vi "TraverseControl.vi"(0 "Mode":T1=enum."Read traverse position", 1 "Route Checking?":bool, 3 "Traverse Name":string, 7 "Model       Roll      Pitch       Yaw (deg)":dbl[](array[numeric]) format="%#.2f", 11 "Position input XYZ":dbl[](array[numeric])=[0.0, 0.0, 0.0] format="%.2f", 13 "Speed Factor":dbl=1.0 min=0.1 max=5.0 format="%.2f", 14 "Backlash Compensation?":bool=TRUE) -> (4 "Position Output XYZ":dbl[](array[numeric]) format="%.2f", 15 "Error String":string)   [LabVIEW 2011]
uses:
  Anemometry/Anemometry Sub Vis/Gen Trav/Trav_mode.ctl
  ~subVIs/GenericDriveCommand.ctl
  ADAM Client/Sub VIs/ADAM Controls/Update_scan_value.ctl
  Anemometry/Anemometry Sub Vis/Globals/Trav_pos_global.vi
  Anemometry/Anemometry Sub Vis/Globals/Preference_global.vi
  ~subVIs/DriveConfigGlobal.vi
  Anemometry/Anemometry Sub Vis/Gen Trav/Route mapping/Route_mapping_global.vi
panel:
  out "Server copy Location":path
  out "Position Steps":dbl[][](array[numeric]) format="%.2f"
  out "Log File":path
  out "Achieved Pos In Eng units of all channels":dbl[](array[numeric]) format="%.2f"
  out "Pulses Positon all channels":dbl[](array[numeric])
  out "Counters Reset?":bool
  # "X                Y                   Z"
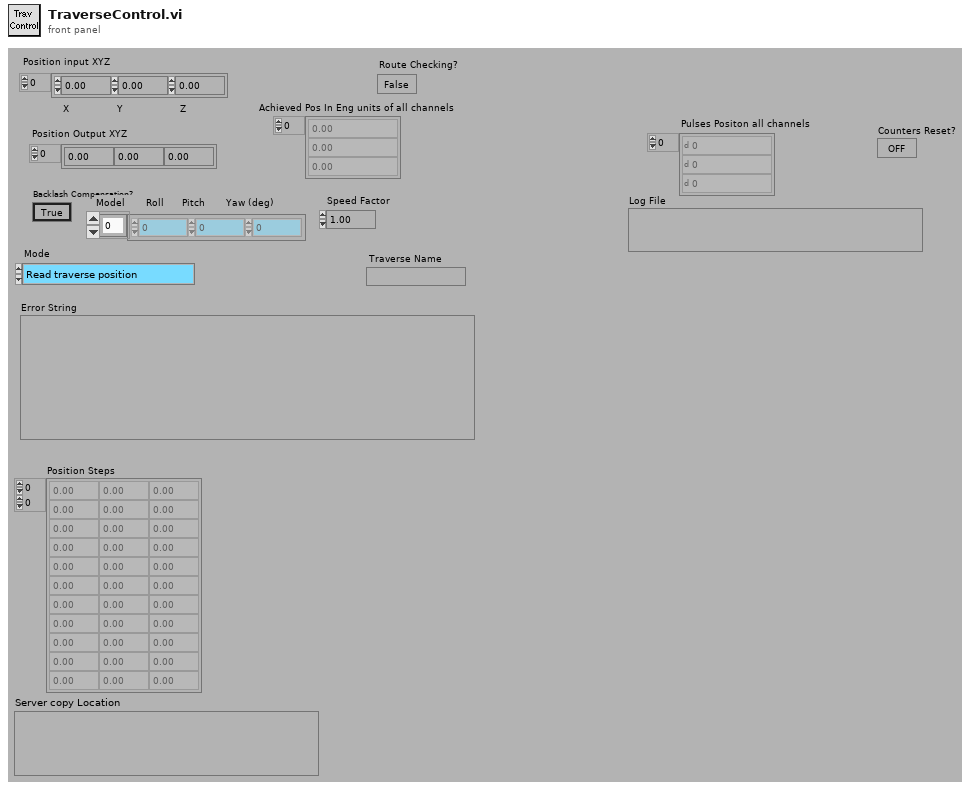
[diagram p1: front panel]
types:
  T1 = typedef "Trav_mode.ctl" = enum16{"Move traverse", "Read traverse position", "Teach Position"}
  T2 = typedef "Tunnel_Coordinates.ctl" = enum16{"Work in Tunnel Coordinates", "Work in Model Coordinates"}
  T3 = typedef "GenericDriveCommand.ctl" = string
  T4 = enum16{"To Traverse Coordinates", "To User Coordinates"}
  T5 = typedef "Update_scan_value.ctl" = cluster{"Channel Name":string, "New Value":dbl}
  T6 = typedef "AxisConfigCluster.ctl" = cluster{"Channel Properties":T7, "Static Drive Configuration":T8}
  T7 = typedef "DriveProperties.ctl" = cluster{"Channel Name":string, "Vel. Default":dbl, "Acc. Default":dbl, "Vel. Max":dbl, "Vel. Min":dbl, "Acc. Max":dbl, "Acc. Min":dbl, "Pulses/unit":dbl, "Address":u8, "Pulse Offset":i32, "Pos Tolerance":dbl, "Pulses/rev":dbl, "Backlash/Eng units":dbl, "Current Pos":dbl, "Ch Status":enum16{"Active", "Offline", "Simulate"}, "Port Name":string, "Axis Transform mode":string, "Metadata Ch Name":string, "Type":string}
  T8 = typedef "DriveStaticConfig.ctl" = cluster{"Correction Gain % (CG)":u16, "Dead Band (DB)":i32, "Dead Band Window (DW)":i32, "Encoder Resolution (ER)":i32, "Step Mode  (FSB)":u16, "Position Maintenance (FSC)":u16, "Stop on Stall (FSD)":u16, "Activate OP1 on stall (FSE)":u16, "Stop on Trigger 3 (FSF)":u16, "OP2 in Deadband (FSG)":u16, "Stall Detect (FSH)":u16, "Limit Disable (LD)":u16, "Motor Resolution (MR)":enum16{"200", "400", "1000", "2000", "4000", "5000", "10000", "12800", "18000", "20000", "21600", "25000", "25400", "25600", "36000", "50000", "278528", "425984", "507904", "614400", "655360", "819200", "1024000"}, "Limit Switch Sense (OSA)":u16, "Home Position (OSB)":u16, "Home Switch Sense (OSC)":u16, "Encoder Z for Home (OSD)":u16, "Reference edge of Home (OSH)":u16, "RS232 Echo Control (SSA)":u16, "Buffer at Limit (SSG)":u16, "Buffer at Stop (SSH)":u16, "Indexer Mode  (FSA)":u16, "Type":string, "ConfigString":string, "De Power Motor":enum16{"TRUE", "FALSE"}}
  T9 = typedef "Box_size.ctl" = cluster{"Max":dbl, "Min":dbl}[]
  T10 = typedef "Exclude_cluster.ctl" = cluster{"Sizes":T9, "Name":string, "Exclude Type":T11}
  T11 = typedef "Exclusion_type.ctl" = enum16{"Exclude completely", "Allow only vertical moves"}
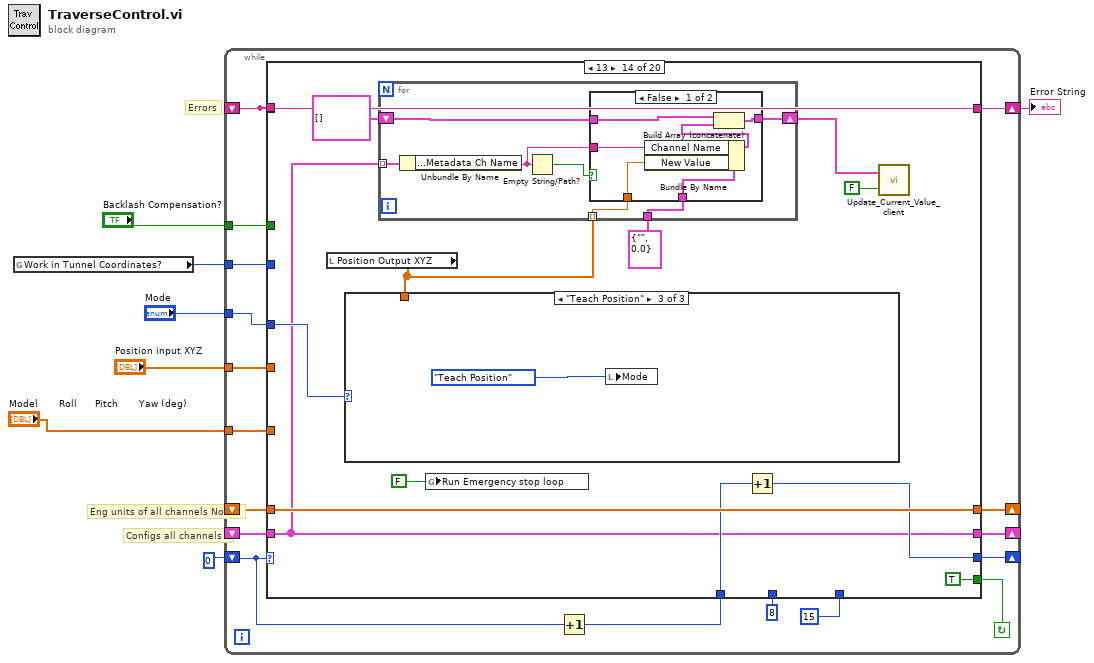
[diagram p0: block diagram]
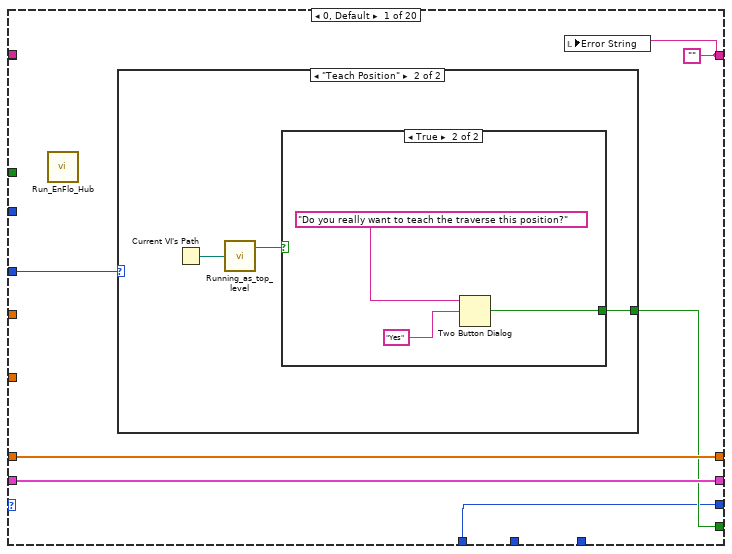
[diagram p2: hidden frame]
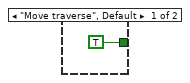
[diagram p3: hidden frame]
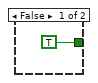
[diagram p4: hidden frame]
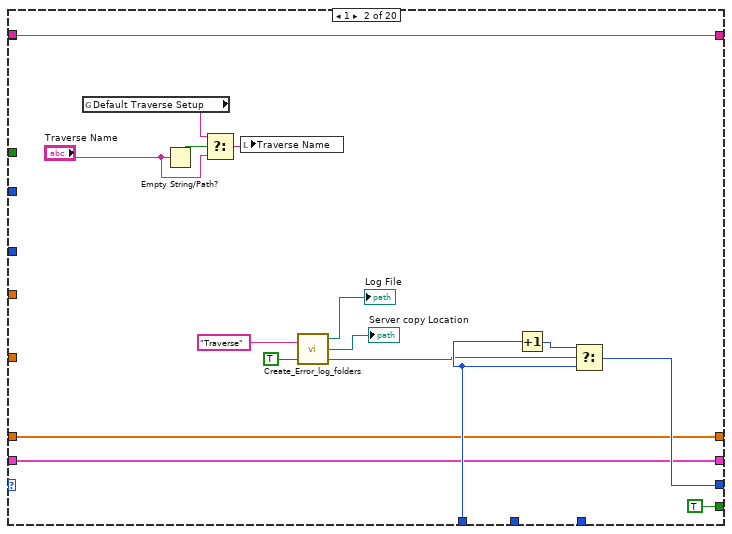
[diagram p5: hidden frame]
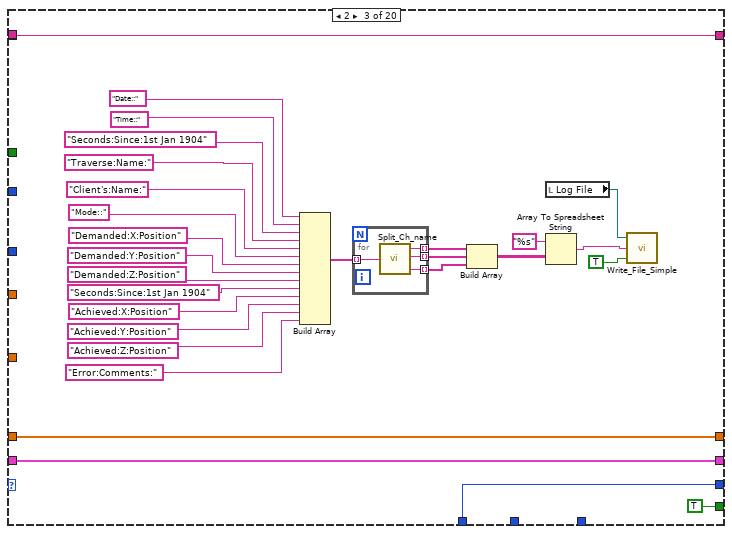
[diagram p6: hidden frame]
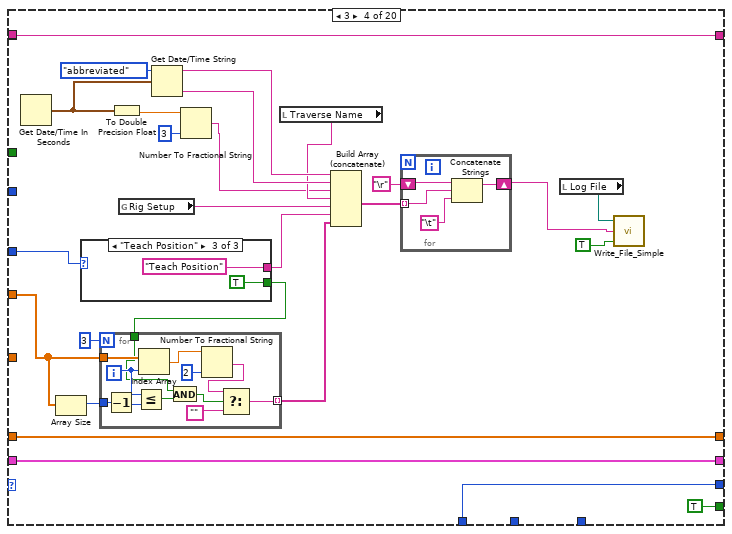
[diagram p7: hidden frame]
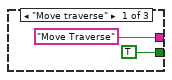
[diagram p8: hidden frame]
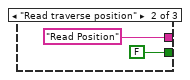
[diagram p9: hidden frame]
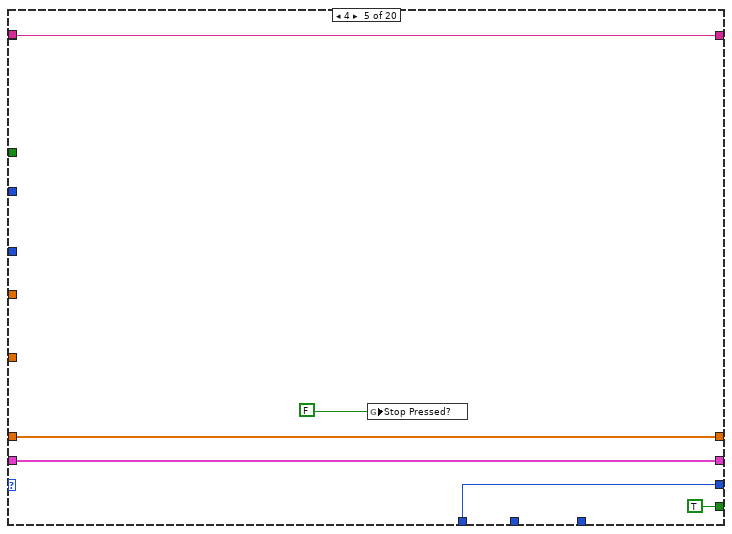
[diagram p10: hidden frame]
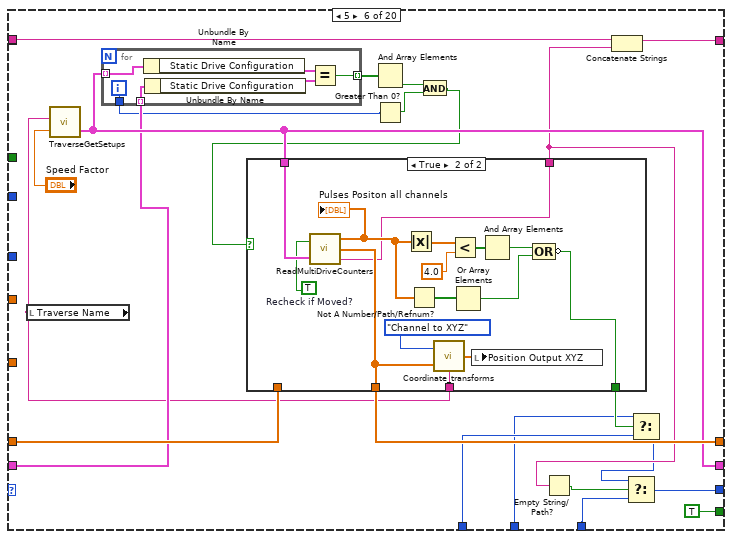
[diagram p11: hidden frame]
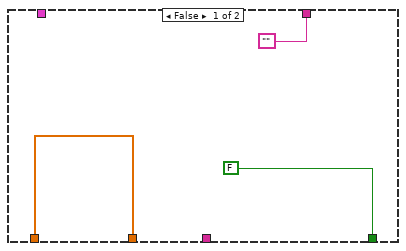
[diagram p12: hidden frame]
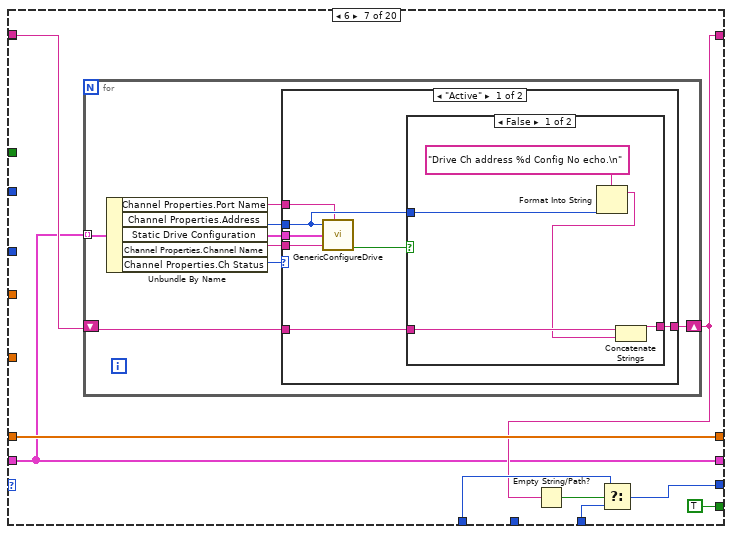
[diagram p13: hidden frame]
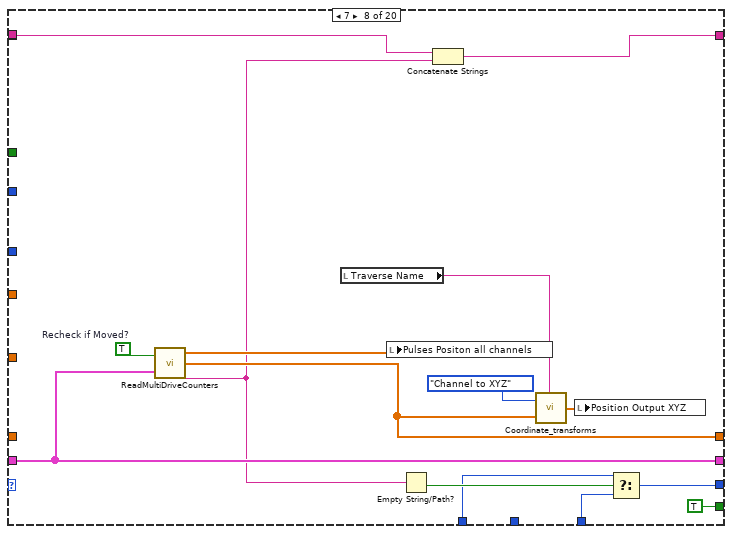
[diagram p16: hidden frame]
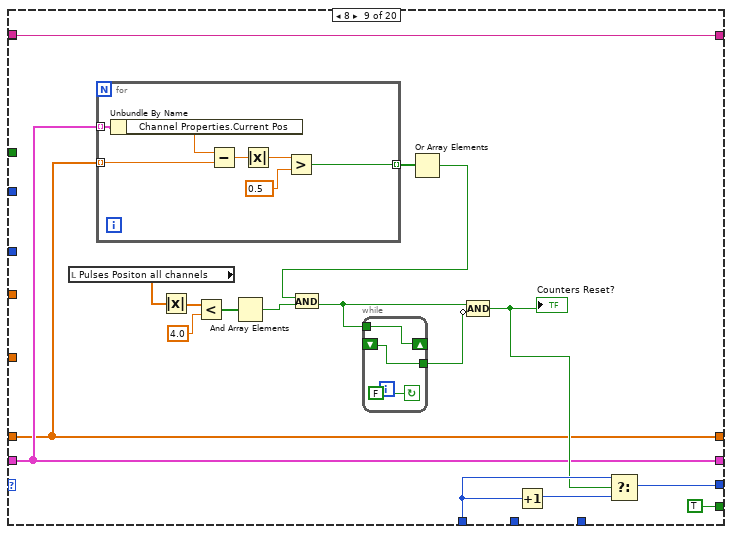
[diagram p17: hidden frame]
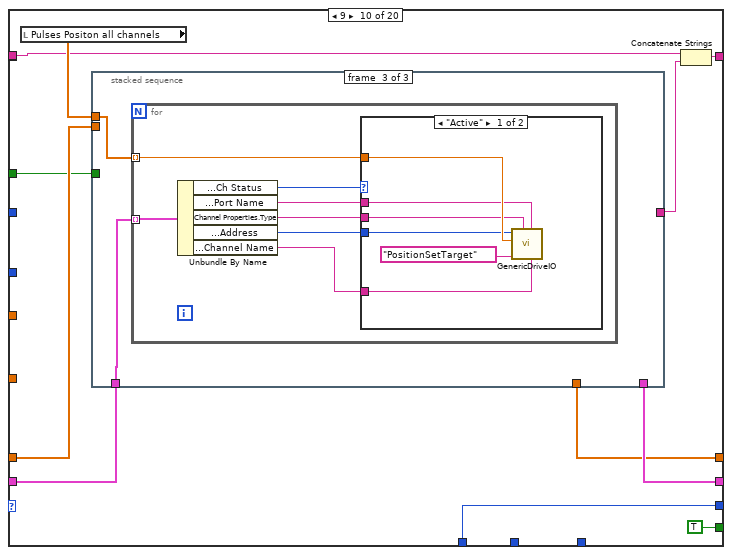
[diagram p18: hidden frame]
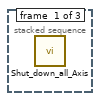
[diagram p19: hidden frame]
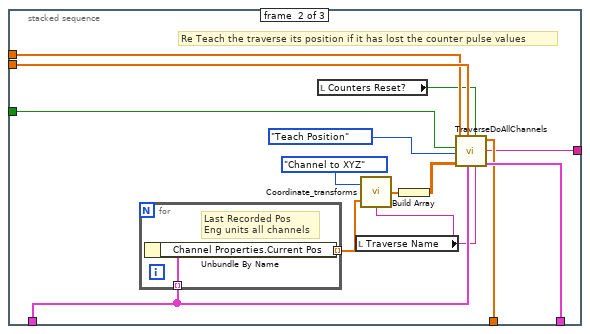
[diagram p20: hidden frame]
diagram:
  # "Errors"
  # "Eng units of all channels Now"
  # "Configs all channels"
  n1 = global read "Trav_pos_global.vi" "Work in Tunnel Coordinates?"() -> (w2:T2)
  n2 = while {
    tunnel: "Backlash Compensation?" -> [w10]
    tunnel: "Position input XYZ" -> [w14]
    shift-left: _ -> [w11]
    shift-right: [w15] -> w5
    shift-left: _ -> [w16]
    shift-right: [w17] -> _
    shift-left: _ -> [w18]
    shift-right: [w19] -> _
    shift-left: 0 -> [w22]
    shift-right: [w20] -> _
    tunnel: "Mode" -> [w24]
    tunnel: "Model       Roll      Pitch       Yaw (deg)" -> [w9]
    tunnel: w2 -> [w8]
    stop <- w23 continue-if-true
    n3 = Increment(x=w22) -> (x+1=w21:i32)
    n4 = case shown="13" w22 {
      tunnel: w24 -> [w30 _ _ w105 _ _ _ _ _ _ w309 _ w373 w380 _ _ _ w453 _ w509]
      tunnel: [w27 TRUE ("T button?") TRUE ("T button?") TRUE ("T button?") TRUE TRUE ("T button?") TRUE ("T button?") TRUE ("T button?") TRUE TRUE TRUE ("T button?") TRUE ("T button?") TRUE TRUE TRUE ("T button?") TRUE ("T button?") TRUE ("T button?") w455 TRUE FALSE] -> w23
      tunnel: w21 -> [w26 w53 w62 w110 w135 w159 w192 w220 w245 w261 w308 w342 w364 w382 w405 w419 w448 w452 w487 w516]
      tunnel: [w26 w51 w62 w110 w135 w142 w191 w218 w243 w261 w307 w343 w364 w381 w405 w417 w448 w451 w487 w516] -> w20
      tunnel: [w28 w48 w64 w112 w137 w157 w187 w232 w239 w270 w305 w345 w357 w379 w407 w431 w450 w458 w485 w514] -> w19
      tunnel: w18 -> [w28 w48 w64 w112 w137 w156 w187 w232 w239 w269 w305 w345 w371 w379 w407 w431 w450 w458 w485 w514]
      tunnel: [w29 w49 w63 w111 w138 w162 w195 w227 w238 w266 w304 w332 w365 w385 w406 w430 w449 w459 w488 w517] -> w17
      tunnel: w16 -> [w29 w49 w63 w111 w138 w161 w195 _ w238 w267 w304 w332 w360 w385 w406 w430 w449 w459 w488 w517]
      tunnel: [w25 w47 w60 w102 w139 w147 w188 w223 w242 w263 w310 w336 w367 w383 w403 w421 w446 w454 w481 w510] -> w15
      tunnel: w11 -> [_ w47 w60 w102 w139 w148 w189 w224 w242 w265 w310 _ w368 w383 w403 w421 w446 w457 w483 w512]
      tunnel: w14 -> [_ _ _ w99 _ _ _ _ _ _ w303 w334 _ _ _ _ _ _ w479 _]
      tunnel: 15 ("f") -> [_ _ _ _ _ w143 w190 w219 _ _ _ w338 _ _ _ _ _ _ _ _]
      tunnel: 8 ("t") -> [_ _ _ _ _ w158 _ _ _ _ _ _ _ _ _ _ _ _ _ _]
      tunnel: w11 -> [_ _ _ _ _ _ _ _ _ _ _ w339 _ _ _ _ _ _ _ _]
      tunnel: w10 -> [_ _ _ _ _ _ _ _ _ w260 _ _ w359 _ _ _ _ _ _ _]
      tunnel: w9 -> [_ _ _ _ _ _ _ _ _ _ _ w319 _ _ _ _ _ _ w480 w507]
      tunnel: w8 -> [_ _ _ _ _ _ _ _ _ _ _ _ _ _ _ _ _ _ w477 w505]
      frame 0, Default {
        w25 = ""
        n5 = call "Run_EnFlo_Hub.vi"() -> ()  [unwired: 8 out]
        n6 = case shown="\"Teach Position\"" w30 {
          tunnel: [TRUE ("T button?") w32] -> w27
          frame "Move traverse", Default {
          }
          frame "Teach Position" {
            n7 = Current VI's Path() -> (path=w34:path)
            n8 = call "Running_as_top_level.vi"("Vi path name"=w34) -> ("Top Level"=w33:bool)  [unwired: 1 out]
            n9 = case shown="True" w33 {
              tunnel: [TRUE ("T button?") w36] -> w32
              frame False {
              }
              frame True {
                n10 = Two Button Dialog(message="Do you really want to teach the traverse this position?", 2:"Yes" ("T button name (\"OK\")")) -> (T button?=w36:bool)  [unwired: 1 out]
              }
            }
          }
        }
        n11 = local write "Error String"(w25) -> ()
      }
      frame 1 {
        n12 = global read "Trav_pos_global.vi" "Default Traverse Setup"() -> (w44:string)
        n13 = Empty String/Path?(string/path="Traverse Name") -> (empty?=w42:bool)
        n14 = Select(t=w44, s=w42, f="Traverse Name") -> (s? t:f=w41:string)
        n15 = local write "Traverse Name"(w41) -> ()
        n16 = call "Create_Error_log_folders.vi"("Per Day Log File?"=TRUE, "Log Filename"="Traverse" ("Input Element")) -> ("exists?"=w45:bool, "Server copy Location"=→"Server copy Location":path, "Local Log File"=→"Log File":path)  [unwired: 1 in]
        n17 = Increment(x=w53) -> (x+1=w52:i32)
        n18 = Select(t=w52, s=w45, f=w53) -> (s? t:f=w51:i32)
      }
      frame 2 {
        n19 = Build Array("Date::", "Time::", "Seconds:Since:1st Jan 1904", "Traverse:Name:", "Client's:Name:", "Mode::", "Demanded:X:Position", "Demanded:Y:Position", "Demanded:Z:Position", "Seconds:Since:1st Jan 1904", "Achieved:X:Position", "Achieved:Y:Position", "Achieved:Z:Position", "Error:Comments:") -> (w67:string[])
        n20 = for {
          tunnel: w67 -> [w86] mode=indexing
          tunnel: [w85] -> w68 mode=indexing
          tunnel: [w84] -> w69 mode=indexing
          tunnel: [w83] -> w70 mode=indexing
          n21 = call "Split_Ch_name.vi"("Ch name"=w86) -> ("Top level"=w85:string, "Middle"=w84:string, "Low level"=w83:string)
        }
        n22 = Build Array(w68, w69, w70) -> (w65:string[][])
        n23 = local read "Log File"() -> (w56:path)
        n24 = Array To Spreadsheet String(array=w65, 3:"%s" ("format string")) -> (spreadsheet string=w57:string)  [unwired: 1 out]
        n25 = call "Write_File_Simple.vi"("append to file? (new file:F)"=TRUE, "character string"=w57, "file path"=w56) -> ()  [unwired: 2 out]
      }
      frame 3 {
        n26 = Get Date/Time In Seconds() -> (seconds since 1Jan1904=w91:timestamp)
        n27 = Array Size(array=w99) -> (size(s)=w100:i32)
        n28 = case shown="\"Teach Position\"" w105 {
          tunnel: ["Move Traverse" "Read Position" "Teach Position"] -> w106
          tunnel: [TRUE FALSE TRUE] -> w96
          frame "Move traverse" {
          }
          frame "Read traverse position" {
          }
          frame "Teach Position" {
          }
        }
        n29 = for {
          N: 3 -> [_]
          tunnel: w99 -> [w124]
          tunnel: w100 -> [w121]
          tunnel: [w117] -> w97 mode=indexing
          tunnel: w96 -> [w113]
          i -> [w119]
          n30 = Decrement(x=w121) -> (x-1=w120:i32)
          n31 = Less Or Equal?(x=w119, y=w120) -> (x <= y?=w115:bool)
          n32 = Index Array(array=w124, index=w119) -> (element=w123:dbl)
          n33 = And(x=w113, y=w115) -> (x .and. y?=w114:bool)
          n34 = Number To Fractional String(number=w123, precision (6)=i16 2) -> (F-format string=w118:string)  [unwired: 2 out]
          n35 = Select(t=w118, s=w114, f="") -> (s? t:f=w117:string)
        }
        n36 = To Double Precision Float(number=w91) -> (double precision float=w90:dbl)
        n37 = global read "Preference_global.vi" "Rig Setup"() -> (w87:string)
        n38 = Get Date/Time String(date format (0)=enum16{"short", "long", "abbreviated"}."abbreviated", seconds (now)=w91) -> (date string=w108:string, time string=w107:string)  [unwired: 1 out]
        n39 = Number To Fractional String(number=w90, precision (6)=i16 3) -> (F-format string=w88:string)  [unwired: 2 out]
        n40 = local read "Traverse Name"() -> (w92:string)
        n41 = Build Array (concatenate)(w108, w107, w88, w92, w87, w106, w97) -> (w103:string[])
        n42 = for {
          shift-right: [w127] -> w93
          shift-left: "\r" -> [w128]
          tunnel: w103 -> [w126] mode=indexing
          n43 = Concatenate Strings(w128, w126, "\t") -> (w127:string)
        }
        n44 = local read "Log File"() -> (w94:path)
        n45 = call "Write_File_Simple.vi"("append to file? (new file:F)"=TRUE, "character string"=w93, "file path"=w94) -> ()  [unwired: 2 out]
      }
      frame 4 {
        n46 = global write "DriveConfigGlobal.vi" "Stop Pressed?"(FALSE) -> ()
      }
      frame 5 {
        n47 = local read "Traverse Name"() -> (w150:string)
        n48 = call "TraverseGetSetups.vi"("Speed Factor"="Speed Factor", "Traverse Name"=w150) -> ("Matched Configurations"=w157:T6[])  [unwired: 1 out]
        n49 = for {
          tunnel: w157 -> [w168] mode=indexing
          tunnel: w156 -> [w167] mode=indexing
          tunnel: [w164] -> w155 mode=indexing
          tunnel: [w163] -> w154
          i -> [w163]
          n50 = Unbundle By Name(w168) -> ("Static Drive Configuration"=w166:T8)
          n51 = Unbundle By Name(w167) -> ("Static Drive Configuration"=w165:T8)
          n52 = Equal?(x=w166, y=w165) -> (x = y?=w164:bool)
        }
        n53 = And Array Elements(Boolean array=w155) -> (logical AND=w152:bool)
        n54 = Greater Than 0?(x=w154) -> (x > 0?=w153:bool)
        n55 = And(x=w152, y=w153) -> (x .and. y?=w151:bool)
        n56 = case shown="True" w151 {
          tunnel: w157 -> [_ w186]
          tunnel: [w171 w176] -> w162
          tunnel: w161 -> [w171 _]
          tunnel: [FALSE w178] -> w160
          tunnel: w150 -> [_ w174]
          tunnel: ["" w172] -> w146
          frame False {
          }
          frame True {
            w173 = TRUE  # Recheck if Moved?
            n57 = call "ReadMultiDriveCounters.vi"("Recheck if Moved?"=w173, "Matched Configurations"=w186) -> ("Pulses"=w181:dbl[], "Eng units"=w176:dbl[], "Error String"=w172:string)
            "Pulses Positon all channels" <- w181
            n58 = Absolute Value(x=w181) -> (abs(x)=w185:dbl[])
            n59 = Not A Number/Path/Refnum?(number/path/refnum=w181) -> (NaN/Path/Refnum?=w180:bool[])
            n60 = call "Coordinate_transforms.vi"("Traverse Name"=w174, "Input"=w176, "Mode"=enum16{"XYZ to Channel", "Channel to XYZ"}."Channel to XYZ") -> ("Output"=w175:dbl[])
            n61 = Less?(x=w185, y=4.0 ("Achieved Position")) -> (x < y?=w183:bool[])
            n62 = Or Array Elements(Boolean array=w180) -> (logical OR=w179:bool)
            n63 = local write "Position Output XYZ"(w175) -> ()
            n64 = And Array Elements(Boolean array=w183) -> (logical AND=w182:bool)
            n65 = Compound Arithmetic op=OR(w182, w179) -> (invert w178:bool)
          }
        }
        n66 = Empty String/Path?(string/path=w146) -> (empty?=w145:bool)
        n67 = Concatenate Strings(w148, w146) -> (w147:string)
        n68 = Select(t=w158, s=w160, f=w159) -> (s? t:f=w144:i32)
        n69 = Select(t=w144, s=w145, f=w143) -> (s? t:f=w142:i32)
      }
      frame 6 {
        n70 = for {
          tunnel: w187 -> [w203] mode=indexing
          shift-right: [w196] -> w188
          shift-left: w189 -> [w197]
          n71 = Unbundle By Name(w203) -> ("Channel Properties.Port Name"=w198:string, "Channel Properties.Address"=w202:u8, "Static Drive Configuration"=w201:T8, "Channel Properties.Channel Name"=w200:string, "Channel Properties.Ch Status"=w199:enum16{"Active", "Offline", "Simulate"})
          n72 = case shown="\"Active\"" w199 {
            tunnel: w202 -> [w208 _]
            tunnel: w201 -> [w210 _]
            tunnel: w200 -> [w209 _]
            tunnel: w198 -> [w207 _]
            tunnel: w197 -> [w205 w217]
            tunnel: [w204 w217] -> w196
            frame "Active" {
              n73 = call "GenericConfigureDrive.vi"("Address"=w208, "Port Name"=w207, "Static Drive Configuration"=w210, "Channel Name"=w209) -> ("Good Echo"=w206:bool)  [unwired: 4 out]
              n74 = case shown="False" w206 {
                tunnel: w208 -> [w215 _]
                tunnel: w205 -> [w213 w216]
                tunnel: [w212 w216] -> w204
                frame False {
                  n75 = Format Into String(format string="Drive Ch address %d Config No echo.\n" ("Format String"), w215) -> (resulting string=w211:string)  [unwired: 2 in, 1 out]
                  n76 = Concatenate Strings(w213, w211) -> (w212:string)
                }
                frame True {
                }
              }
            }
            frame "Offline", Default {
            }
          }
        }
        n77 = Empty String/Path?(string/path=w188) -> (empty?=w193:bool)
        n78 = Select(t=w192, s=w193, f=w190) -> (s? t:f=w191:i32)
      }
      frame 7 {
        w225 = TRUE  # Recheck if Moved?
        n79 = call "ReadMultiDriveCounters.vi"("Recheck if Moved?"=w225, "Matched Configurations"=w232) -> ("Pulses"=w230:dbl[], "Eng units"=w227:dbl[], "Error String"=w221:string)
        n80 = local read "Traverse Name"() -> (w226:string)
        n81 = local write "Pulses Positon all channels"(w230) -> ()
        n82 = Empty String/Path?(string/path=w221) -> (empty?=w222:bool)
        n83 = Concatenate Strings(w224, w221) -> (w223:string)
        n84 = call "Coordinate_transforms.vi"("Traverse Name"=w226, "Input"=w227, "Mode"=enum16{"XYZ to Channel", "Channel to XYZ"}."Channel to XYZ") -> ("Output"=w228:dbl[])
        n85 = local write "Position Output XYZ"(w228) -> ()
        n86 = Select(t=w220, s=w222, f=w219) -> (s? t:f=w218:i32)
      }
      frame 8 {
        n87 = local read "Pulses Positon all channels"() -> (w233:dbl[])
        n88 = for {
          tunnel: w239 -> [w259] mode=indexing
          tunnel: w238 -> [w257] mode=indexing
          tunnel: [w253] -> w236 mode=indexing
          n89 = Unbundle By Name(w259) -> ("Channel Properties.Current Pos"=w258:dbl)
          n90 = Subtract(x=w258, y=w257) -> (x-y=w256:dbl)
          n91 = Absolute Value(x=w256) -> (abs(x)=w255:dbl)
          n92 = Greater?(x=w255, y=0.5) -> (0:w253:bool)
        }
        n93 = Absolute Value(x=w233) -> (abs(x)=w249:dbl[])
        n94 = Less?(x=w249, y=4.0 ("Achieved Position")) -> (x < y?=w247:bool[])
        n95 = And Array Elements(Boolean array=w247) -> (logical AND=w237:bool)
        n96 = Or Array Elements(Boolean array=w236) -> (logical OR=w235:bool)
        n97 = And(x=w235, y=w237) -> (x .and. y?=w234:bool)
        n98 = while {
          tunnel: [w251] -> w241
          tunnel: w234 -> [w252]
          shift-left: _ -> [w251]
          shift-right: [w252] -> _
          stop <- FALSE continue-if-true
        }
        n99 = Compound Arithmetic op=AND(w234, invert w241) -> (w240:bool)
        "Counters Reset?" <- w240
        n100 = Increment(x=w245) -> (x+1=w244:i32)
        n101 = Select(t=w245, s=w240, f=w244) -> (s? t:f=w243:i32)
      }
      frame 9 {
        n102 = local read "Pulses Positon all channels"() -> (w268:dbl[])
        n103 = stacked-sequence {
          tunnel: w268 -> [_ w276 w287]
          tunnel: [_ w284 _] -> w270
          tunnel: w267 -> [_ w283 _]
          tunnel: [_ w282 _] -> w266
          tunnel: w269 -> [_ w278 w288]
          tunnel: [_ w281 _] -> w264
          tunnel: w260 -> [_ w272 _]
          frame #0 {
            n104 = call "Shut_down_all_Axis.vi"() -> ()  [unwired: 1 out]
          }
          frame #1 {
            # "Re Teach the traverse its position if it has lost the counter pulse values"
            n105 = for {
              tunnel: [w286] -> w277 mode=indexing
              tunnel: w278 -> [w285] mode=indexing
              # "Last Recorded Pos\nEng units all channels"
              n106 = Unbundle By Name(w285) -> ("Channel Properties.Current Pos"=w286:dbl)
            }
            n107 = local read "Counters Reset?"() -> (w274:bool)
            n108 = local read "Traverse Name"() -> (w273:string)
            n109 = call "Coordinate_transforms.vi"("Traverse Name"=w273, "Input"=w277, "Mode"=enum16{"XYZ to Channel", "Channel to XYZ"}."Channel to XYZ") -> ("Output"=w279:dbl[])
            n110 = Build Array(w279) -> (w271:dbl[][])
            n111 = call "TraverseDoAllChannels.vi"("Traverse Name"=w273, "Counters Reset?"=w274, "Matched Configurations all Channels In"=w278, "Current Pos In Eng units of all channels"=w283, "Position Steps"=w271, "Mode"=Trav_mode."Teach Position", "Backlash Compensation?"=w272, "Current Pulses positions for all channels"=w276) -> ("Matched Configurations Out"=w284:T6[], "Error String"=w281:string, "Achieved Pos In Eng units of all channels"=w282:dbl[])  [unwired: 1 out]
          }
          frame #2 {
            n112 = for {
              tunnel: w288 -> [w295] mode=indexing
              tunnel: w287 -> [w294] mode=indexing
              n113 = Unbundle By Name(w295) -> ("Channel Properties.Ch Status"=w293:enum16{"Active", "Offline", "Simulate"}, "Channel Properties.Port Name"=w292:string, "Channel Properties.Type"=w291:string, "Channel Properties.Address"=w290:u8, "Channel Properties.Channel Name"=w289:string)
              n114 = case shown="\"Active\"" w293 {
                tunnel: w294 -> [w301 _]
                tunnel: w292 -> [w300 _]
                tunnel: w291 -> [w299 _]
                tunnel: w290 -> [w298 _]
                tunnel: w289 -> [w297 _]
                frame "Active" {
                  n115 = call "GenericDriveIO.vi"("GenericDriveCommand"=T3 "PositionSetTarget", "Channel Name"=w297, "Numeric Value"=w301, "Address"=w298, "Type"=w299, "Port Name"=w300) -> ()  [unwired: 1 in, 5 out]
                }
                frame "Offline", Default {
                }
              }
            }
          }
        }
        n116 = Concatenate Strings(w265, w264) -> (w263:string)
      }
      frame 10 {
        n117 = Build Array(w303) -> (w302:dbl[][])
        n118 = local write "Position Steps"(w302) -> ()
        n119 = case shown="\"Read traverse position\", Default" w309 {
          tunnel: w308 -> [w311 w318]
          tunnel: [w313 w317] -> w307
          frame "Move traverse" {
            n120 = Increment(x=w311) -> (x+1=w312:i32)
            n121 = case shown="True" "Route Checking?" {
              tunnel: [w315 w316] -> w313
              tunnel: w312 -> [w315 _]
              tunnel: w311 -> [_ w316]
              frame False {
              }
              frame True {
              }
            }
          }
          frame "Read traverse position", Default {
            n122 = Increment(x=w318) -> (x+1=w317:i32)
          }
        }
      }
      frame 11 {
        w325 = 0.1  # Reduce by
        w331 = TRUE  # Full Check
        n123 = global read "Route_mapping_global.vi" "Probe Volume"() -> (w324:T9)
        n124 = local read "Traverse Name"() -> (w333:string)
        n125 = for {
          tunnel: w324 -> [w352] mode=indexing
          tunnel: [w351] -> w323 mode=indexing
          tunnel: w325 -> [w346]
          n126 = Unbundle By Name(w352) -> ("Max"=w350:dbl, "Min"=w348:dbl)
          n127 = Subtract(x=w350, y=w346) -> (x-y=w349:dbl)
          n128 = Add(x=w346, y=w348) -> (x+y=w347:dbl)
          n129 = Bundle By Name(cluster=w352, "Max"=w349, "Min"=w347) -> (w351:cluster{"Max":dbl, "Min":dbl})
        }
        n130 = global read "Route_mapping_global.vi" "Entire Space"() -> (w326:T9)
        n131 = global read "Route_mapping_global.vi" "Exclude Array"() -> (w327:T10[])
        n132 = call "Coordinate_transforms.vi"("Traverse Name"=w333, "Input"=w332, "Mode"=enum16{"XYZ to Channel", "Channel to XYZ"}."Channel to XYZ") -> ("Output"=w321:dbl[])
        n133 = call "Coordinate_rotation.vi"("Model       Roll      Pitch       Yaw (deg)"=w319, "Input Position"=w321, "Mode"=T4."To User Coordinates") -> ("Output Position"=w320:dbl[])  [unwired: 2 in, 1 out]
        n134 = call "Coordinate_rotation.vi"("Model       Roll      Pitch       Yaw (deg)"=w319, "Input Position"=w334, "Mode"=T4."To User Coordinates") -> ("Output Position"=w340:dbl[])  [unwired: 2 in, 1 out]
        n135 = call "Check_Traverse_move.vi"("Current position"=w320, "Traverse Name"=w333, "Full Check"=w331, "New Position"=w340, "Model       Roll      Pitch       Yaw (deg)"=w319, "Probe Volume"=w323, "Entire Space"=w326, "Exclude Array"=w327) -> ("Steps"=w330:dbl[][], "Error Comments"=w328:string)  [unwired: 6 out]
        n136 = Empty String/Path?(string/path=w328) -> (empty?=w337:bool)
        n137 = for {
          tunnel: w330 -> [w355] mode=indexing
          tunnel: [w354] -> w329 mode=indexing
          tunnel: w319 -> [w353]
          n138 = call "Coordinate_rotation.vi"("Model       Roll      Pitch       Yaw (deg)"=w353, "Input Position"=w355, "Mode"=T4."To Traverse Coordinates") -> ("Output Position"=w354:dbl[])  [unwired: 2 in, 1 out]
        }
        "Position Steps" <- w329
        n139 = Select(t=w342, s=w337, f=w338) -> (s? t:f=w343:i32)
        n140 = Concatenate Strings(w339, w328) -> (w336:string)
      }
      frame 12 {
        w362 = FALSE  # Counters Reset?
        n141 = local read "Pulses Positon all channels"() -> (w372:dbl[])
        n142 = local read "Traverse Name"() -> (w361:string)
        n143 = local read "Position Steps"() -> (w358:dbl[][])
        n144 = call "TraverseDoAllChannels.vi"("Traverse Name"=w361, "Counters Reset?"=w362, "Matched Configurations all Channels In"=w371, "Current Pos In Eng units of all channels"=w360, "Position Steps"=w358, "Mode"=w373, "Backlash Compensation?"=w359, "Current Pulses positions for all channels"=w372) -> ("Matched Configurations Out"=w357:T6[], "Error String"=w366:string, "Achieved Pos In Eng units of all channels"=w365:dbl[])  [unwired: 1 out]
        "Achieved Pos In Eng units of all channels" <- w365
        n145 = call "Coordinate_transforms.vi"("Traverse Name"=w361, "Input"=w365, "Mode"=enum16{"XYZ to Channel", "Channel to XYZ"}."Channel to XYZ") -> ("Output"=→"Position Output XYZ":dbl[])
        n146 = Concatenate Strings(w368, w366) -> (w367:string)
      }
      frame 13 {
        n147 = local read "Position Output XYZ"() -> (w377:dbl[])
        n148 = case shown="\"Teach Position\"" w380 {
          tunnel: w377 -> [_ w401 _]
          frame "Move traverse" {
          }
          frame "Read traverse position" {
            n149 = local write "Position input XYZ"(w401) -> ()
          }
          frame "Teach Position" {
            n150 = local write "Mode"(Trav_mode."Teach Position" ("Mode")) -> ()
          }
        }
        n151 = for {
          tunnel: w379 -> [w393] mode=indexing
          tunnel: T5 {"Channel Name"="", "New Value"=0.0} ("Update Scan Value Cluster") -> [w392]
          tunnel: w377 -> [w390] mode=indexing
          shift-right: [w388] -> w375
          shift-left: T5[] [] -> [w389]
          n152 = Unbundle By Name(w393) -> ("Channel Properties.Metadata Ch Name"=w391:string)
          n153 = Empty String/Path?(string/path=w391) -> (empty?=w387:bool)
          n154 = case shown="False" w387 {
            tunnel: w392 -> [w399 _]
            tunnel: w391 -> [w398 _]
            tunnel: w390 -> [w397 _]
            tunnel: w389 -> [w395 w400]
            tunnel: [w394 w400] -> w388
            frame False {
              n155 = Bundle By Name(cluster=w399, "Channel Name"=w398, "New Value"=w397) -> (w396:T5)
              n156 = Build Array (concatenate)(w395, w396) -> (w394:T5[])
            }
            frame True {
            }
          }
        }
        n157 = global write "DriveConfigGlobal.vi" "Run Emergency stop loop"(FALSE ("Run Emergency stop loop")) -> ()
        n158 = Increment(x=w382) -> (x+1=w381:i32)
        n159 = call "Update_Current_Value_client.vi"("Don't Bother with check?"=FALSE, "Update array in"=w375) -> ()
      }
      frame 14 {
      }
      frame 15 {
        n160 = local read "Position Output XYZ"() -> (w425:dbl[])
        n161 = Array Size(array=w425) -> (size(s)=w424:i32)
        n162 = Get Date/Time In Seconds() -> (seconds since 1Jan1904=w416:timestamp)
        n163 = for {
          N: 3 -> [_]
          tunnel: w425 -> [w445]
          tunnel: w424 -> [w442]
          tunnel: [w437] -> w423 mode=indexing
          i -> [w440]
          n164 = Decrement(x=w442) -> (x-1=w441:i32)
          n165 = Less Or Equal?(x=w440, y=w441) -> (x <= y?=w439:bool)
          n166 = Index Array(array=w445, index=w440) -> (element=w444:dbl)
          n167 = Number To Fractional String(number=w444, precision (6)=i16 2) -> (F-format string=w438:string)  [unwired: 2 out]
          n168 = Select(t=w438, s=w439, f="") -> (s? t:f=w437:string)
        }
        n169 = To Double Precision Float(number=w416) -> (double precision float=w409:dbl)
        n170 = Number To Fractional String(number=w409, precision (6)=i16 3) -> (F-format string=w408:string)  [unwired: 2 out]
        n171 = call "Remove_unprintable_Char.vi"("Input String"=w421) -> ("Output String"=w422:string)
        n172 = Build Array (concatenate)(w408, w423, w422) -> (w427:string[])
        n173 = local read "Route Checking?"() -> (w420:bool)
        n174 = for {
          shift-right: [w434] -> w413
          shift-left: "" -> [w435]
          tunnel: w427 -> [w433] mode=indexing
          n175 = Concatenate Strings(w435, w433, "\t") -> (w434:string)
        }
        n176 = Increment(x=w419) -> (x+1=w418:i32)
        n177 = local read "Server copy Location"() -> (w411:path)
        n178 = local read "Log File"() -> (w414:path)
        n179 = Select(t=w418, s=w420, f=w419) -> (s? t:f=w417:i32)
        n180 = call "Write_File_Simple.vi"("append to file? (new file:F)"=TRUE, "character string"=w413, "file path"=w414) -> ("file path Out"=w412:path)  [unwired: 1 out]
        n181 = call "Updated_File_Copy.vi"("Target Path"=w411, "Source Path"=w412) -> ()  [unwired: 2 out]
      }
      frame 16 {
      }
      frame 17 {
        n182 = local read "Position Output XYZ"() -> (w460:dbl[])
        n183 = local read "Counters Reset?"() -> (w461:bool)
        n184 = Index Array(array=w460, index=2) -> (element=w466:dbl)
        n185 = Index Array(array=w460, index=0) -> (element=w468:dbl)
        n186 = Index Array(array=w460, index=1) -> (element=w467:dbl)
        n187 = Format Into String(format string="X= %.2f\tY= %.2f\tZ= %.2f" ("Format String"), w468, w467, w466) -> (resulting string=w469:string)  [unwired: 2 in, 1 out]
        n188 = case shown="\"Read traverse position\"" w453 {
          tunnel: w452 -> [w473 w475]
          tunnel: [w473 w474] -> w451
          frame "Move traverse", Default {
          }
          frame "Read traverse position" {
            n189 = Increment(x=w475) -> (x+1=w474:i32)
          }
        }
        n190 = Select(t="\nThe traverse was probably powered down since the last move. Its position has now been retaught and now all should be well.", s=w461, f="") -> (s? t:f=w462:string)
        n191 = call "Write_out_serial_log.vi"("Header message"=w469) -> ()
        n192 = Concatenate Strings(w457, w462) -> (w454:string)
        n193 = Empty String/Path?(string/path=w454) -> (empty?=w456:bool)
        n194 = Not(x=w456) -> (.not. x?=w455:bool)
      }
      frame 18 {
        # "Add demanded position"
        n195 = case shown="\"Work in Model Coordinates\"" w477 {
          tunnel: w480 -> [_ w495]
          tunnel: w479 -> [w490 w494]
          tunnel: [w490 w492] -> w478
          tunnel: [" (Tunnel Coordinates)" " (Model Coordinates)"] -> w476
          frame "Work in Tunnel Coordinates" {
          }
          frame "Work in Model Coordinates" {
            n196 = call "Coordinate_rotation.vi"("Model       Roll      Pitch       Yaw (deg)"=w495, "Input Position"=w494, "Mode"=T4."To User Coordinates") -> ("Output Position"=w492:dbl[])  [unwired: 2 in, 1 out]
          }
        }
        n197 = for {
          tunnel: w485 -> [w503] mode=indexing
          shift-right: [w498] -> w482
          shift-left: "\nDem Pos " -> [w501]
          tunnel: w478 -> [w496] mode=indexing
          n198 = Unbundle By Name(w503) -> ("Channel Properties.Channel Name"=w502:string)
          n199 = call "Split_Ch_name.vi"("Ch name"=w502) -> ("Low level"=w500:string)  [unwired: 2 out]
          n200 = Format Into String(format string="%s=%.1f, " ("Format String"), w500, w496) -> (resulting string=w497:string)  [unwired: 2 in, 1 out]
          n201 = Concatenate Strings(w501, w497) -> (w498:string)
        }
        n202 = Concatenate Strings(w483, w482, w476) -> (w481:string)
      }
      frame 19 {
        # "Add Achieved Position"
        n203 = local read "Position Output XYZ"() -> (w504:dbl[])
        n204 = case shown="\"Work in Model Coordinates\"" w505 {
          tunnel: w507 -> [_ w521]
          tunnel: [w518 w520] -> w506
          tunnel: w504 -> [w518 w519]
          frame "Work in Tunnel Coordinates" {
          }
          frame "Work in Model Coordinates" {
            n205 = call "Coordinate_rotation.vi"("Model       Roll      Pitch       Yaw (deg)"=w521, "Input Position"=w519, "Mode"=T4."To User Coordinates") -> ("Output Position"=w520:dbl[])  [unwired: 2 in, 1 out]
          }
        }
        n206 = for {
          tunnel: w514 -> [w533] mode=indexing
          shift-right: [w528] -> w511
          shift-left: "\nAchieved Pos " -> [w531]
          tunnel: w506 -> [w526] mode=indexing
          n207 = Unbundle By Name(w533) -> ("Channel Properties.Channel Name"=w532:string)
          n208 = call "Split_Ch_name.vi"("Ch name"=w532) -> ("Low level"=w530:string)  [unwired: 2 out]
          n209 = Format Into String(format string="%s=%.1f, " ("Format String"), w530, w526) -> (resulting string=w527:string)  [unwired: 2 in, 1 out]
          n210 = Concatenate Strings(w531, w527) -> (w528:string)
        }
        n211 = case shown="\"Move traverse\"" w509 {
          tunnel: ["When requesting a move." "When reading position." "When teaching position."] -> w508
          frame "Move traverse" {
          }
          frame "Read traverse position" {
          }
          frame "Teach Position" {
          }
        }
        n212 = Concatenate Strings(w512, w511, w508) -> (w510:string)
      }
    }
  }
  "Error String" <- w5
